vi "Create Bundles.vi"(1 "Time":dbl[](array[numeric]), 2 "Frequency":dbl[](array[numeric]), 3 "Data":dbl[](array[numeric])) -> (8 "Bundled Array":T1(array[cluster]))   [LabVIEW 2014, in "Melody Extraction.lvlib"]
uses:
  Melody Extraction.lvlib
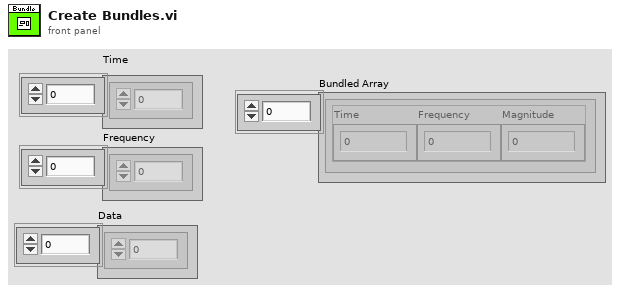
[diagram p1: front panel]
types:
  T1 = cluster{"Time":dbl, "Frequency":dbl, "Magnitude":dbl}[]
  T2 = cluster{"Time":dbl, "Frequency":dbl, "Magnitude":dbl}
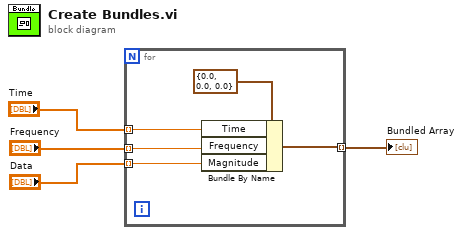
[diagram p0: block diagram]
diagram:
  n1 = for {
    tunnel: "Time" -> [w9] mode=indexing
    tunnel: "Data" -> [w6] mode=indexing
    tunnel: [w8] -> w1 mode=indexing
    tunnel: "Frequency" -> [w7] mode=indexing
    n2 = Bundle By Name(cluster=T2 {"Time"=0.0, "Frequency"=0.0, "Magnitude"=0.0} ("Cluster"), "Time"=w9, "Frequency"=w7, "Magnitude"=w6) -> (w8:T2)
  }
  "Bundled Array" <- w1
